vi "host.vi"() -> ()   [LabVIEW 2020]
uses:
  <vilib>/Analysis/7linalg.llb/Real Transpose Matrix.vi
  <vilib>/Utility/file.llb/Write Delimited Spreadsheet (DBL).vi
  <vilib>/Analysis/NI_AALPro.lvlib
panel:
  in  "ms per read sample":dbl
  out "Waveform Graph":dbl[][](graph)
  out "y predict values":dbl[](array[numeric])
  in  "y predict save":path
  out "time":dbl
  out "t":dbl[][](array[numeric])
  out "y waveform":cluster{"Numeric":dbl, "Double":dbl}(graph)
  in  "stop":bool
  out "iteration":dbl
  out "max iteration":dbl
  in  "t data filepath":path
  in  "y data filepath":path
  out "y":dbl[][](array[numeric])
  out "size":dbl
  in  "X data filepath":path
  out "X":dbl[][](array[numeric])
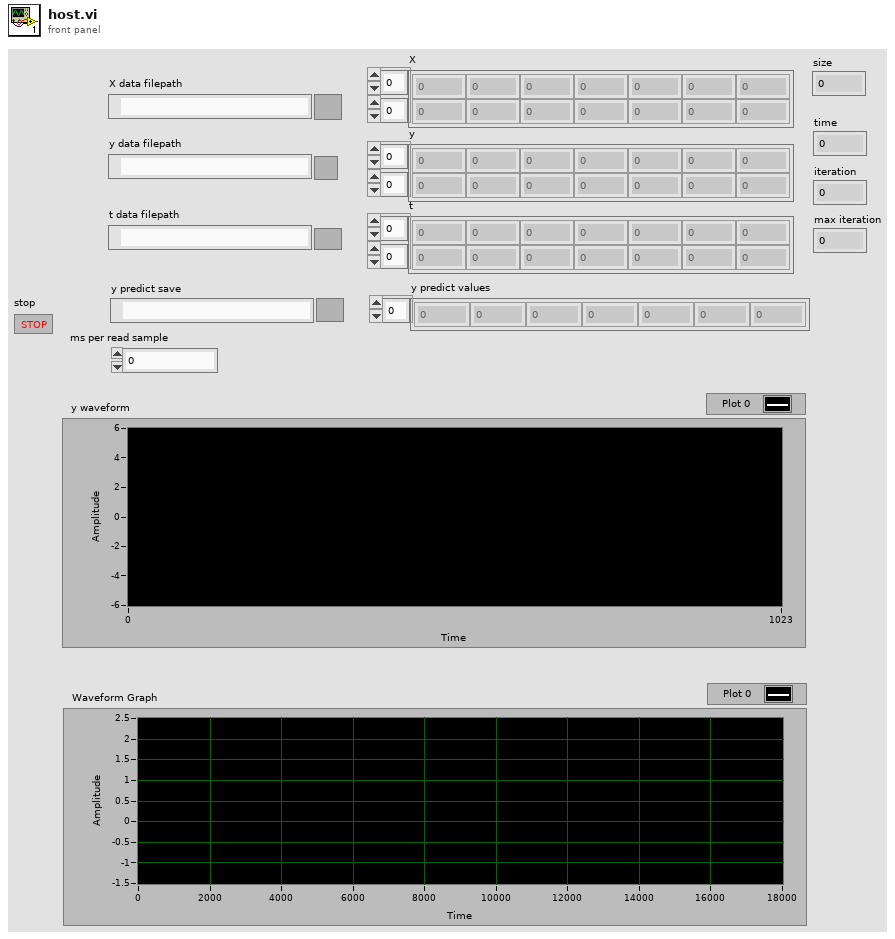
[diagram p1: front panel]
types:
  T1 = typedef "NI_Matrix.lvlib/RealMatrix.ctl" = dbl[][]
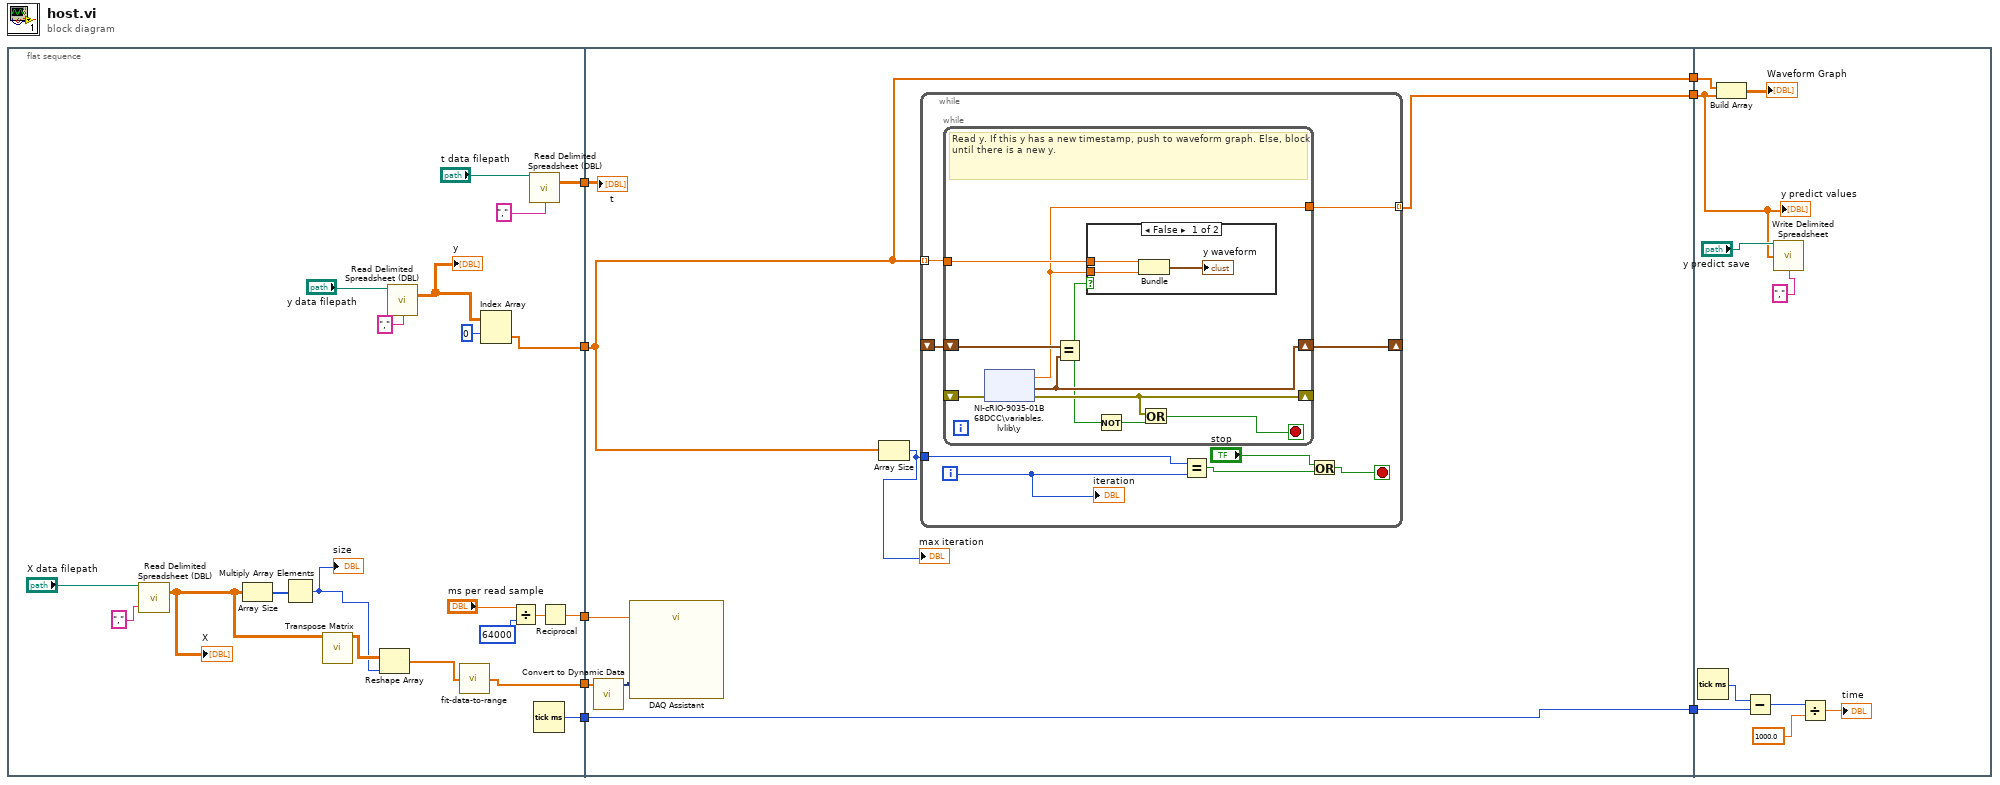
[diagram p0: block diagram]
diagram:
  n1 = flat-sequence {
    tunnel: [w27] -> w8
    tunnel: [w20] -> w7
    tunnel: [w19] -> w6
    tunnel: [w14] -> w2
    tunnel: [w11] -> w1
    tunnel: w8 -> [w37]
    tunnel: w7 -> [w33]
    tunnel: w6 -> [w35]
    tunnel: [w35] -> w5
    tunnel: [w34] -> w4
    tunnel: [w33] -> w3
    tunnel: w2 -> [w32]
    tunnel: w1 -> [w30]
    tunnel: w5 -> [w67]
    tunnel: w4 -> [w60]
    tunnel: w3 -> [w63]
    frame #0 {
      n2 = call <vilib>:"Read Delimited Spreadsheet (DBL).vi"("file path (dialog if empty)"="X data filepath", "delimiter (\\t)"=",") -> ("all rows"=w13:dbl[][])  [unwired: 8 in, 5 out]
      "X" <- w13
      n3 = Array Size(array=w13) -> (size(s)=w18:i32[])
      n4 = Multiply Array Elements(1:w18) -> (0:w16:i32)
      "size" <- w16
      n5 = call-poly <vilib>:"Transpose Matrix.vi"("Input Matrix"=w13) -> ("Matrix Transpose"=w17:T1)  [unwired: 9 in, 1 out]
      n6 = Reshape Array(w17, w16) -> (w15:dbl[])
      n7 = call <vilib>:"Read Delimited Spreadsheet (DBL).vi"("file path (dialog if empty)"="y data filepath", "delimiter (\\t)"=",") -> ("all rows"=w25:dbl[][])  [unwired: 8 in, 5 out]
      "y" <- w25
      n8 = call "fit-data-to-range.vi"("in"=w15) -> ("out"=w14:dbl[])
      n9 = Index Array(array=w25, index (row)=0) -> (element=w20:dbl[])  [unwired: 1 in]
      n10 = Divide(x="ms per read sample", y=64000) -> (x/y=w12:dbl)
      n11 = call <vilib>:"Read Delimited Spreadsheet (DBL).vi"("file path (dialog if empty)"="t data filepath", "delimiter (\\t)"=",") -> ("all rows"=w27:dbl[][])  [unwired: 8 in, 5 out]
      n12 = Tick Count (ms)() -> (millisecond timer value=w19:u32)
      n13 = Reciprocal(x=w12) -> (1/x=w11:dbl)
    }
    frame #1 {
      n14 = call "Convert to Dynamic Data"("Array"=w32) -> ("Dynamic Data Type"=w31:dynamicdata)  [unwired: 3 in]
      n15 = call "DAQ Assistant"("data"=w31, "rate"=w30) -> ()  [unwired: 15 in, 3 out]
      n16 = Array Size(array=w33) -> (size(s)=w36:i32)
      "max iteration" <- w36
      n17 = while {
        tunnel: w33 -> [w46] mode=indexing
        tunnel: [w43] -> w34 mode=indexing
        shift-right: [w45] -> _
        shift-left: _ -> [w44]
        tunnel: w36 -> [w42]
        i -> [w38]
        stop <- w40 stop-if-true
        n18 = while {
          shift-right: [w54] -> w45
          shift-left: w44 -> [w53]
          shift-right: [w52] -> _
          shift-left: _ -> [w55]
          tunnel: w46 -> [w49]
          tunnel: [w48] -> w43
          stop <- w47 stop-if-true
          # "Read y. If this y has a new timestamp, push to waveform graph. Else, block until there is a new y."
          n19 = shared-variable "NI-cRIO-9035-01B68DCC\\variables.lvlib\\y"(error in=w55) -> (w48:dbl, error out=w52:errorcluster, w54:timestamp)
          n20 = Equal?(x=w53, y=w54) -> (x = y?=w50:bool)
          n21 = case shown="False" w50 {
            tunnel: w49 -> [w57 _]
            tunnel: w48 -> [w56 _]
            frame False {
              n22 = Bundle("Numeric"=w57, "Double"=w56) -> (→"y waveform":cluster{"Numeric":dbl, "Double":dbl})  [unwired: 1 in]
            }
            frame True {
            }
          }
          n23 = Not(x=w50) -> (.not. x?=w51:bool)
          n24 = Or(x=w52, y=w51) -> (x .or. y?=w47:bool)
        }
        n25 = Equal?(x=w42, y=w38) -> (x = y?=w39:bool)
        n26 = Or(x="stop", y=w39) -> (x .or. y?=w40:bool)
        "iteration" <- w38
      }
      "t" <- w37
    }
    frame #2 {
      n27 = Tick Count (ms)() -> (millisecond timer value=w68:u32)
      n28 = Build Array(w63, w60) -> (→"Waveform Graph":dbl[][])
      n29 = Subtract(x=w68, y=w67) -> (x-y=w66:u32)
      n30 = call-poly <vilib>:"Write Delimited Spreadsheet.vi"("file path (dialog if empty)"="y predict save", "1D data"=w60, "delimiter (\\t)"=",") -> ()  [unwired: 11 in, 2 out]
      n31 = Divide(x=w66, y=1000.0) -> (x/y=→"time":dbl)
      "y predict values" <- w60
    }
  }
